vi "Read object name.vi"(8 "error in (no error)":errorcluster, 11 "SP in":refnum<class "Save messages PGserver.lvclass">) -> (0 "error out":errorcluster, 2 "object name":string, 3 "SP out":refnum<class "Save messages PGserver.lvclass">)   [LabVIEW 2019, in "Save messages PGserver.lvclass"]
uses:
  Save messages PGserver.lvclass
  Save messages PGserver.lvclass/Save messages PGserver.ctl
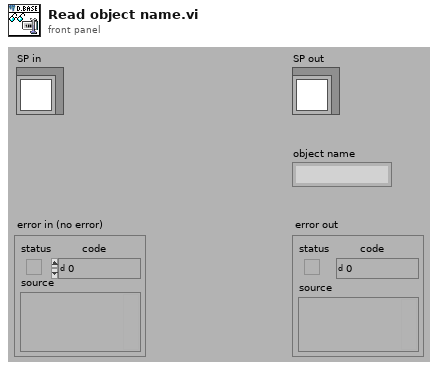
[diagram p1: front panel]
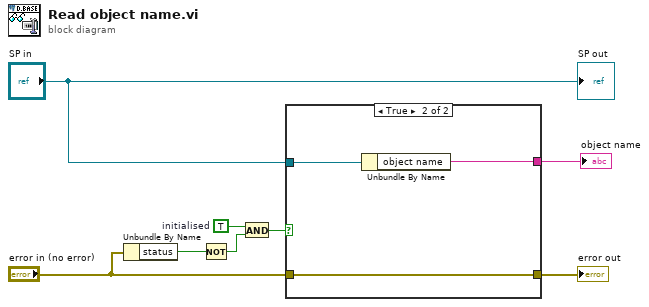
[diagram p0: block diagram]
diagram:
  w3 = TRUE  # initialised
  n1 = Unbundle By Name("error in (no error)") -> ("status"=w6:bool)
  n2 = Not(x=w6) -> (.not. x?=w5:bool)
  n3 = And(x=w3, y=w5) -> (x .and. y?=w7:bool)
  n4 = case shown="True" w7 {
    tunnel: [w9 w11] -> w8
    tunnel: "SP in" -> [_ w12]
    tunnel: "error in (no error)" -> [w9 w11]
    tunnel: [_ w10] -> w1
    frame False {
    }
    frame True {
      n5 = Unbundle By Name(w12) -> ("object name"=w10:string)
    }
  }
  "error out" <- w8
  "object name" <- w1
  "SP out" <- "SP in"
